vi "Numeric Analog Panel.vi"() -> ()   [LabVIEW 2020, in "VolatusGUI.lvlib" / "Telemetry Command Module.lvclass"]
uses:
  Telemetry Command Module.lvclass
  Telemetry Command Module.lvclass/Telemetry Command Module.ctl
panel:
  in  "Value":T1
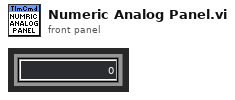
[diagram p1: front panel]
types:
  T1 = cluster{"Color":u32, "Value":dbl, "Backdrop":bool}
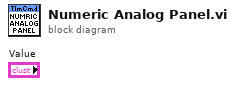
[diagram p0: block diagram]
diagram:
